vi "DP811A DVR.vi"(8 "error in (no error)":errorcluster, 10 "write buffer":string, 11 "VISA resource name":refnum<visa-resource-name>) -> (0 "Power":dbl, 1 "error out":errorcluster, 2 "read buffer":string, 3 "Value":dbl, 4 "Current":dbl, 6 "Voltage":dbl)   [LabVIEW 2025, in "Interface Functions.lvlib"]
uses:
  Interface Functions.lvlib
  <vilib>/Instr/_visa.llb/VISA Open Access Mode.ctl
  80e2d14e-0af9-4134-9fdb-927d146bfa2f.vi
  <vilib>/Utility/error.llb/Trim Whitespace One-Sided.vi
panel:
  out "Retries":i32
  out "read return count":u32
  out "write return count":u32
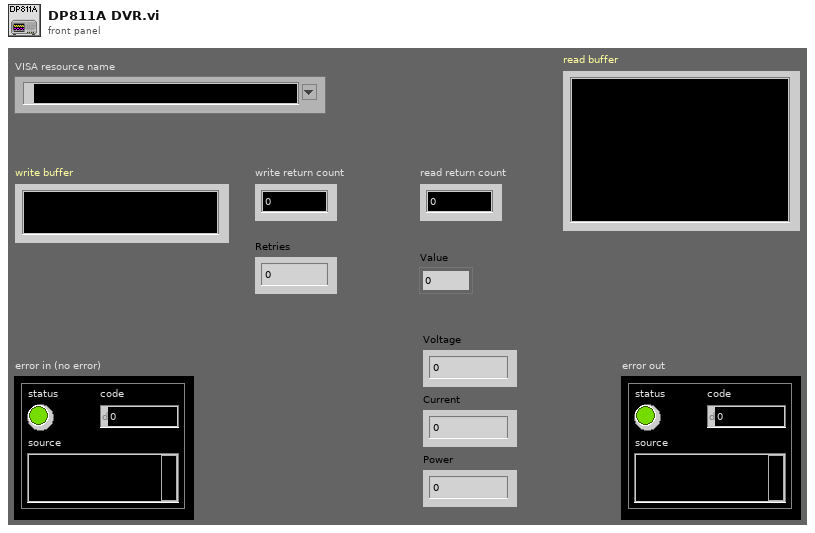
[diagram p1: front panel]
types:
  T1 = typedef "VISA Open Access Mode.ctl" = u32
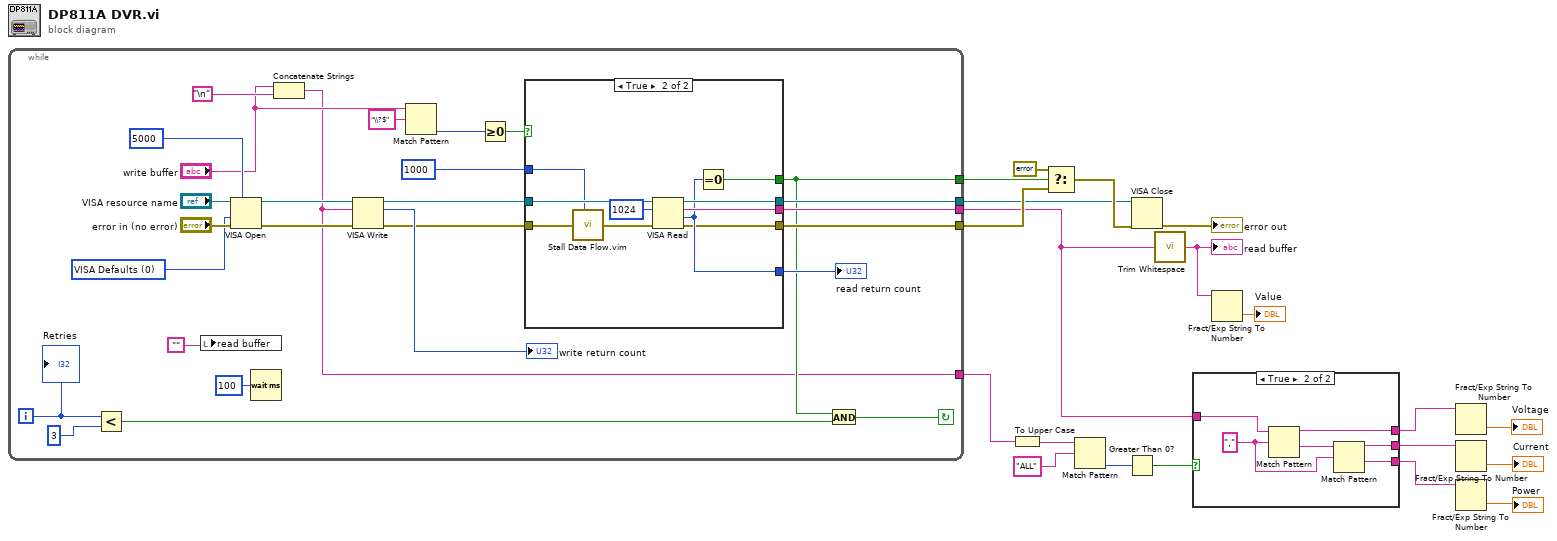
[diagram p0: block diagram]
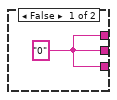
[diagram p2: hidden frame]
diagram:
  n1 = while {
    tunnel: [w34] -> w17
    tunnel: [w26] -> w16
    tunnel: [w33] -> w15
    tunnel: [w30] -> w7
    tunnel: [w21] -> w10
    i -> [w28]
    stop <- w24 continue-if-true
    w45 = T1 0 items=["VISA Defaults"=0, "Exclusive Lock"=1, "Load Configured Settings"=4] ("Access Mode")
    n2 = Less?(x=w28, y=3) -> (x < y?=w25:bool)
    n3 = local write "read buffer"("") -> ()
    n4 = VISA Open(timeout (0)=u32 5000 ("VISA Open timeout (0)"), access mode=w45, error in (no error)="error in (no error)", VISA resource name="VISA resource name") -> (VISA resource name=w42:refnum<visa-resource-name>, error out=w41:errorcluster)  [unwired: 1 in]
    n5 = Wait (ms)(milliseconds to wait=u32 100) -> ()  [unwired: 1 out]
    n6 = Concatenate Strings("write buffer", "\n") -> (w21:string)
    n7 = VISA Write(VISA resource name=w42, write buffer=w21, error in (no error)=w41) -> (VISA resource name out=w35:refnum<visa-resource-name>, return count=→"write return count":u32, error out=w31:errorcluster)
    n8 = Match Pattern(string="write buffer", regular expression="\\?$") -> (offset past match=w38:i32)  [unwired: 1 in, 3 out]
    n9 = Greater Or Equal To 0?(x=w38) -> (x >= 0?=w37:bool)
    n10 = case shown="True" w37 {
      tunnel: w35 -> [w49 w59]
      tunnel: w31 -> [w48 w50]
      tunnel: [w49 w57] -> w33
      tunnel: [_ w56] -> w30
      tunnel: [_ w55] -> w29
      tunnel: [w48 w54] -> w34
      tunnel: [_ w53] -> w26
      tunnel: u32 1000 ("milliseconds to wait") -> [_ w52]
      frame False {
      }
      frame True {
        n11 = call "Stall Data Flow.vim"("value in"=w50, "milliseconds to wait"=w52) -> ("value out"=w51:errorcluster)  [unwired: 1 out]
        n12 = VISA Read(VISA resource name=w59, byte count=u32 1024, error in (no error)=w51) -> (VISA resource name out=w57:refnum<visa-resource-name>, read buffer=w56:string, return count=w55:u32, error out=w54:errorcluster)
        n13 = Equal To 0?(x=w55) -> (x = 0?=w53:bool)
      }
    }
    "read return count" <- w29
    n14 = And(x=w26, y=w25) -> (x .and. y?=w24:bool)
    "Retries" <- w28
  }
  n15 = To Upper Case(1:w10) -> (0:w12:string)
  n16 = Select(t=errorcluster {"status"=FALSE, "code"=0, "source"=""}, s=w16, f=w17) -> (s? t:f=w18:errorcluster)
  n17 = Match Pattern(string=w12, regular expression="ALL") -> (offset past match=w9:i32)  [unwired: 1 in, 3 out]
  n18 = Greater Than 0?(x=w9) -> (x > 0?=w8:bool)
  n19 = VISA Close(VISA resource name=w15, error in (no error)=w18) -> (error out=→"error out":errorcluster)
  n20 = call <vilib>:"Trim Whitespace.vi"("string"=w7) -> ("trimmed string"=w13:string)  [unwired: 1 in]
  "read buffer" <- w13
  n21 = case shown="True" w8 {
    tunnel: w7 -> [_ w65]
    tunnel: [w60 w63] -> w6
    tunnel: [w60 w62] -> w5
    tunnel: [w60 w61] -> w4
    frame False {
      w60 = "0" ("read buffer")
    }
    frame True {
      w64 = "," ("regular expression")
      n22 = Match Pattern(string=w65, regular expression=w64) -> (before substring=w63:string, after substring=w66:string)  [unwired: 1 in, 2 out]
      n23 = Match Pattern(string=w66, regular expression=w64) -> (before substring=w62:string, after substring=w61:string)  [unwired: 1 in, 2 out]
    }
  }
  n24 = Fract/Exp String To Number(string=w13) -> (number=→"Value":dbl)  [unwired: 3 in, 1 out]
  n25 = Fract/Exp String To Number(string=w6) -> (number=→"Voltage":dbl)  [unwired: 3 in, 1 out]
  n26 = Fract/Exp String To Number(string=w5) -> (number=→"Current":dbl)  [unwired: 3 in, 1 out]
  n27 = Fract/Exp String To Number(string=w4) -> (number=→"Power":dbl)  [unwired: 3 in, 1 out]
